vi "Write User Event.vi"   [LabVIEW 2014]
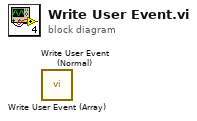
[diagram p0: block diagram]
diagram:
  n1 = call "Write User Event (Array).vi"() -> ()  [unwired: 10 in, 2 out]
  n2 = call "Write User Event (Normal).vi"() -> ()  [unwired: 10 in, 2 out]
